vi "Test Vectors (SHA-1).vi"() -> (3 "All Vectors passed":bool)   [LabVIEW 2013]
uses:
  SHA-1.lvclass
  SHA-1.lvlib
panel:
  out "1 million character message":bool
  out "String tests":bool[](array[boolean])
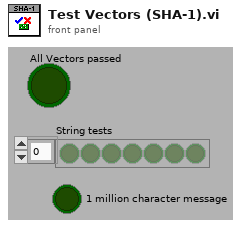
[diagram p1: front panel]
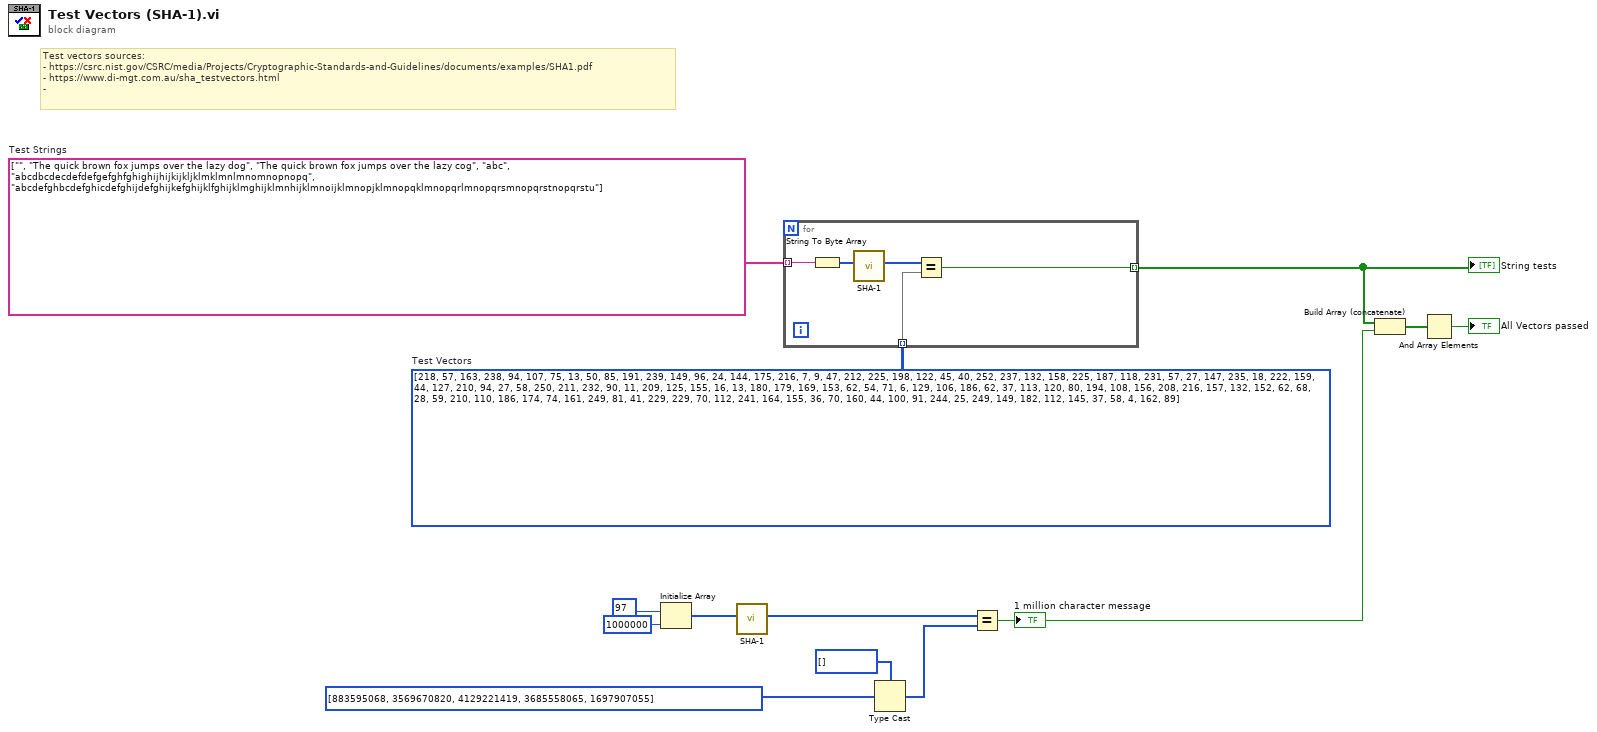
[diagram p0: block diagram]
diagram:
  w13 = string[] ["", "The quick brown fox jumps over the lazy dog", "The quick brown fox jumps over the lazy cog", "abc", "abcdbcdecdefdefgefghfghighijhijkijkljklmklmnlmnomnopnopq", "abcdefghbcdefghicdefghijdefghijkefghijklfghijklmghijklmnhijklmnoijklmnopjklmnopqklmnopqrlmnopqrsmnopqrstnopqrstu"]  # Test Strings
  w9 = u8[][] [[218, 57, 163, 238, 94, 107, 75, 13, 50, 85, 191, 239, 149, 96, 24, 144, 175, 216, 7, 9], [47, 212, 225, 198, 122, 45, 40, 252, 237, 132, 158, 225, 187, 118, 231, 57, 27, 147, 235, 18], [222, 159, 44, 127, 210, 94, 27, 58, 250, 211, 232, 90, 11, 209, 125, 155, 16, 13, 180, 179], [169, 153, 62, 54, 71, 6, 129, 106, 186, 62, 37, 113, 120, 80, 194, 108, 156, 208, 216, 157], [132, 152, 62, 68, 28, 59, 210, 110, 186, 174, 74, 161, 249, 81, 41, 229, 229, 70, 112, 241], [164, 155, 36, 70, 160, 44, 100, 91, 244, 25, 249, 149, 182, 112, 145, 37, 58, 4, 162, 89]]  # Test Vectors
  # "Test vectors sources:\n- https://csrc.nist.gov/CSRC/media/Projects/Cryptographic-Standards-and-Guidelines/documents/examples/SHA1.pdf\n- https://www.di-mgt.com.au/sha_testvectors.html\n-"
  n1 = Initialize Array(u8 97 ("Numeric"), 1000000 ("dimension size")) -> (w10:u8[])
  n2 = call "SHA-1.vi"("data"=w10) -> ("SHA-1 hash"=w8:u8[])  [unwired: 10 in]
  n3 = for {
    tunnel: w13 -> [w18] mode=indexing
    tunnel: w9 -> [w17] mode=indexing
    tunnel: [w16] -> w4 mode=indexing
    n4 = String To Byte Array(string=w18) -> (unsigned byte array=w15:u8[])
    n5 = call "SHA-1.vi"("data"=w15) -> ("SHA-1 hash"=w14:u8[])  [unwired: 10 in]
    n6 = Equal?(x=w14, y=w17) -> (x = y?=w16:bool)
  }
  "String tests" <- w4
  n7 = Type Cast(type=u8[] [], x=u32[] [883595068, 3569670820, 4129221419, 3685558065, 1697907055]) -> (*(type *) &x=w5:u8[])
  n8 = Equal?(x=w8, y=w5) -> (x = y?=w3:bool)
  "1 million character message" <- w3
  n9 = Build Array (concatenate)(w4, w3) -> (w2:bool[])
  n10 = And Array Elements(Boolean array=w2) -> (logical AND=→"All Vectors passed":bool)
